vi "Zoom picture.vi"(10 "error in (no error)":errorcluster, 11 "Picture in":refnum<vi>) -> (2 "error out":errorcluster, 3 "Picture out":refnum<vi>)   [LabVIEW 2014]
doc: "Zooms and pans the picture contol to fit the image."
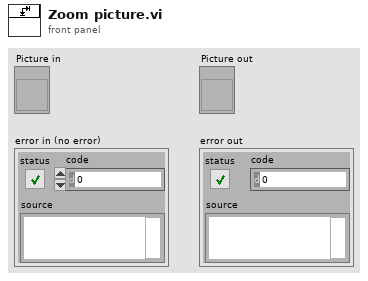
[diagram p1: front panel]
types:
  T1 = typedef "LVBoundsTypeDef.ctl" = cluster{"Width":u32, "Height":u32}
  T2 = typedef "imagedata.ctl" = cluster{"image type":i32, "image depth":i32, "image":u8[], "mask":u8[], "colors":u32[], "Rectangle":cluster{"left":i16, "top":i16, "right":i16, "bottom":i16}}
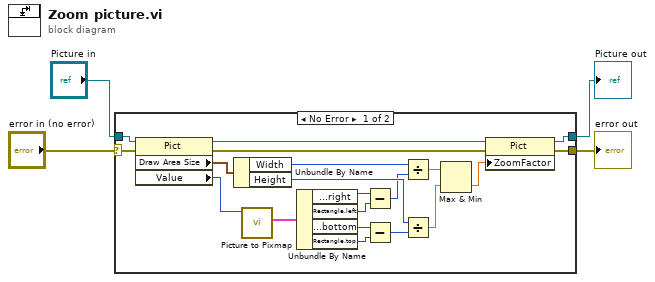
[diagram p0: block diagram]
diagram:
  n1 = case shown="No Error" "error in (no error)" {
    selector: "error in (no error)" -> [w22 w26]
    tunnel: [w24 w25] -> w4
    tunnel: [w23 w26] -> w3
    tunnel: "Picture in" -> [w21 w25]
    frame No Error {
      n2 = property on="Property Node" class="Pict"(reference=w21, error in=w22) -> (reference out=w17:refnum<vi>, error out=w18:errorcluster, "Draw Area Size"=w16:T1, "Value"=w20:picture)
      n3 = Unbundle By Name(w16) -> ("Width"=w10:u32, "Height"=w13:u32)
      n4 = call <vilib>:"Picture to Pixmap.vi"("picture"=w20) -> ("image data"=w19:T2)  [unwired: 9 in, 1 out]
      n5 = Unbundle By Name(w19) -> ("Rectangle.right"=w14:i16, "Rectangle.left"=w15:i16, "Rectangle.bottom"=w7:i16, "Rectangle.top"=w6:i16)
      n6 = Subtract(x=w14, y=w15) -> (x-y=w9:i16)
      n7 = Subtract(x=w7, y=w6) -> (x-y=w5:i16)
      n8 = Divide(x=w10, y=w9) -> (x/y=w12:dbl)
      n9 = Divide(x=w13, y=w5) -> (x/y=w11:dbl)
      n10 = Max & Min(x=w12, y=w11) -> (min(x,y)=w8:dbl)  [unwired: 1 out]
      n11 = property on="Property Node" class="Pict"(reference=w17, error in=w18, "ZoomFactor"=w8) -> (reference out=w24:refnum<vi>, error out=w23:errorcluster)
    }
    frame Error {
    }
  }
  "Picture out" <- w4
  "error out" <- w3
